vi "autonSample.vi"(0 "Auton Array":dbl[][](array[numeric]), 5 "MeasuredHeading":dbl, 9 "EncoderDistance":dbl) -> (4 "Left Drive":dbl(knob) scale=-1.0..1.0, 6 "Right Drive":dbl(knob) scale=-1.0..1.0, 10 "Turret Rotation":dbl, 14 "Feeder motor":dbl, 15 "Shooter motor output":dbl)   [LabVIEW 2011]
uses:
  Robot Global Data.vi
  <vilib>/addons/control/pid/NI_PID_pid.lvlib
  <vilib>/addons/control/pid/pid.llb/PID (DBL).vi
panel:
  out "Tzero":i64
  out "AccumDist":dbl
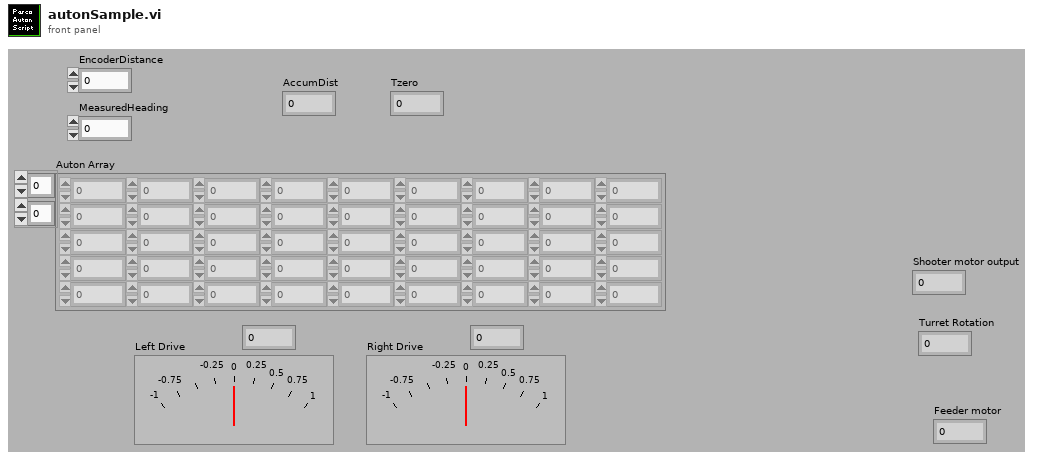
[diagram p1: front panel]
types:
  T1 = cluster{"proportional gain (Kc)":dbl, "integral time (Ti, min)":dbl, "derivative time (Td, min)":dbl}
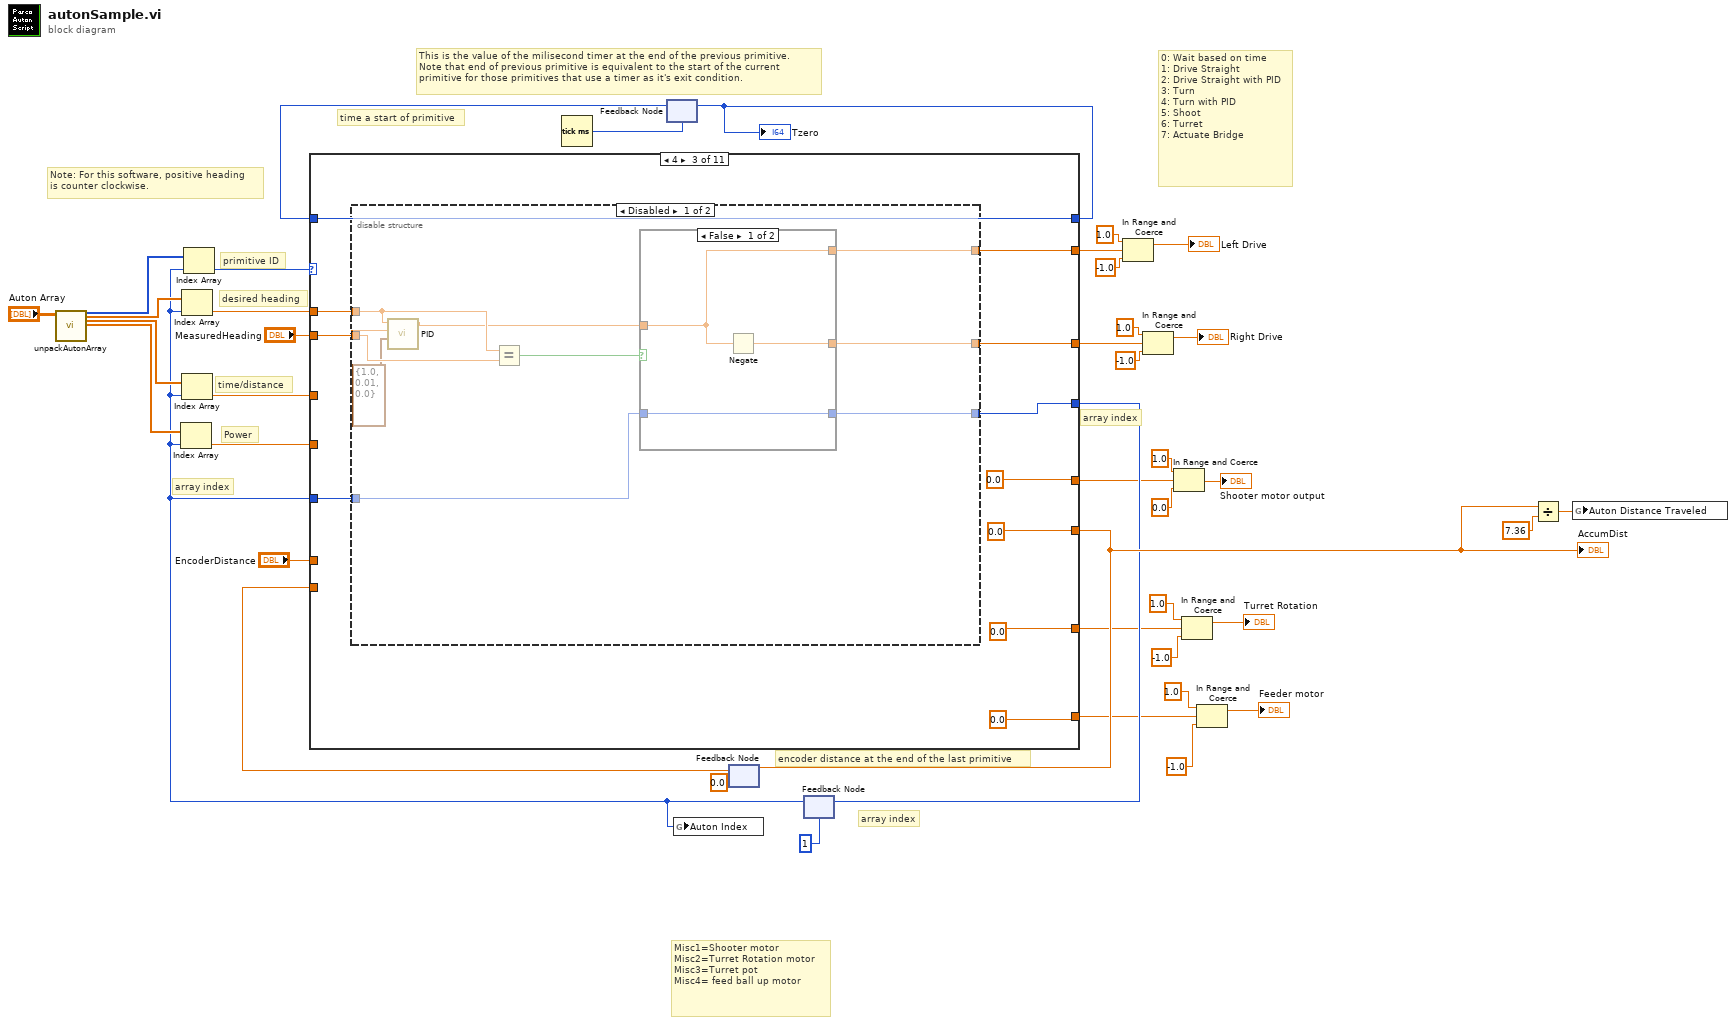
[diagram p0: block diagram]
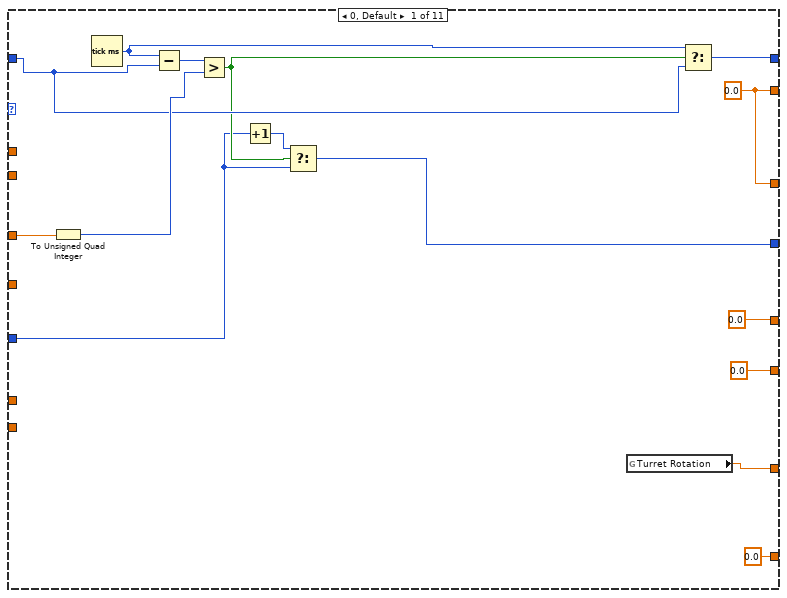
[diagram p2: hidden frame]
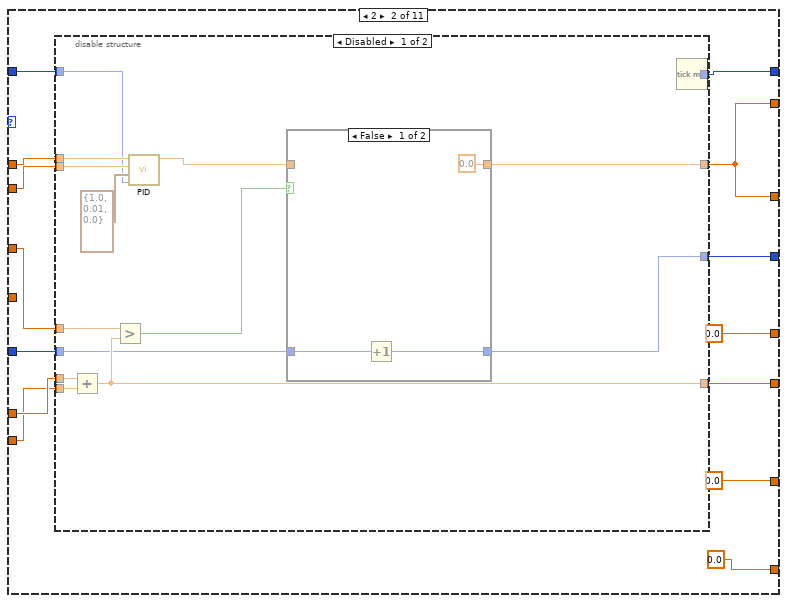
[diagram p3: hidden frame]
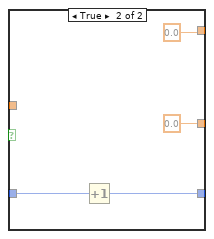
[diagram p6: hidden frame]
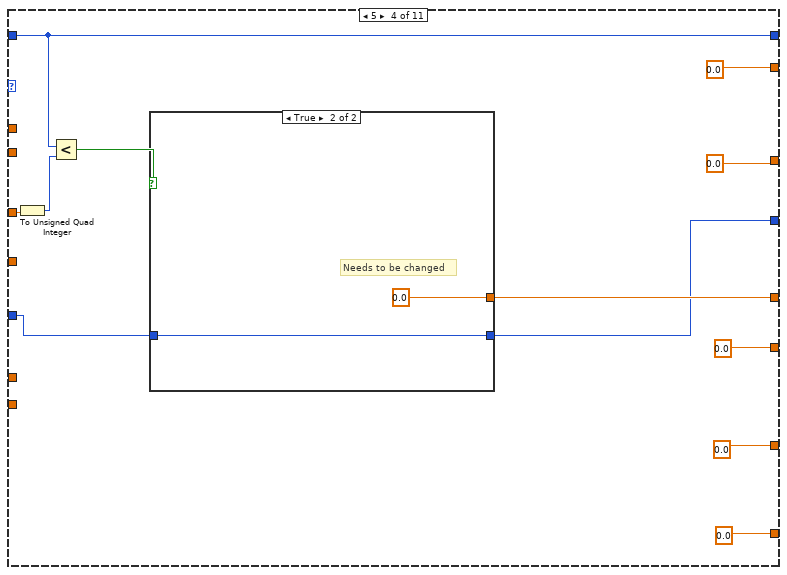
[diagram p8: hidden frame]
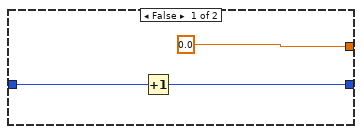
[diagram p9: hidden frame]
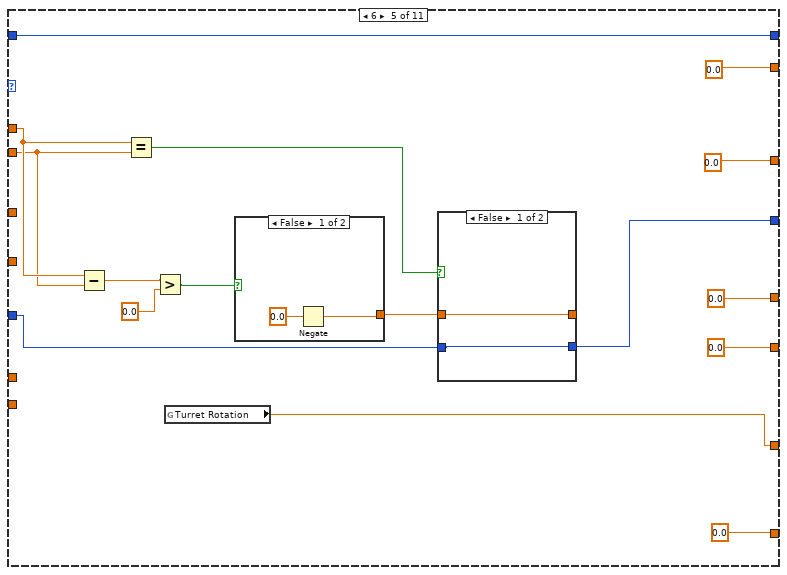
[diagram p10: hidden frame]
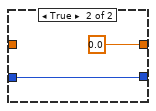
[diagram p11: hidden frame]
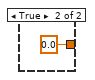
[diagram p12: hidden frame]
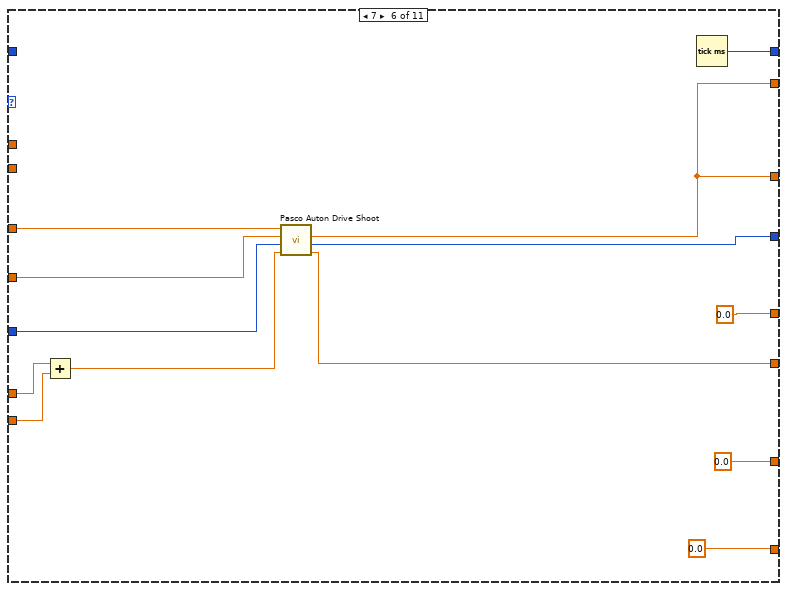
[diagram p13: hidden frame]
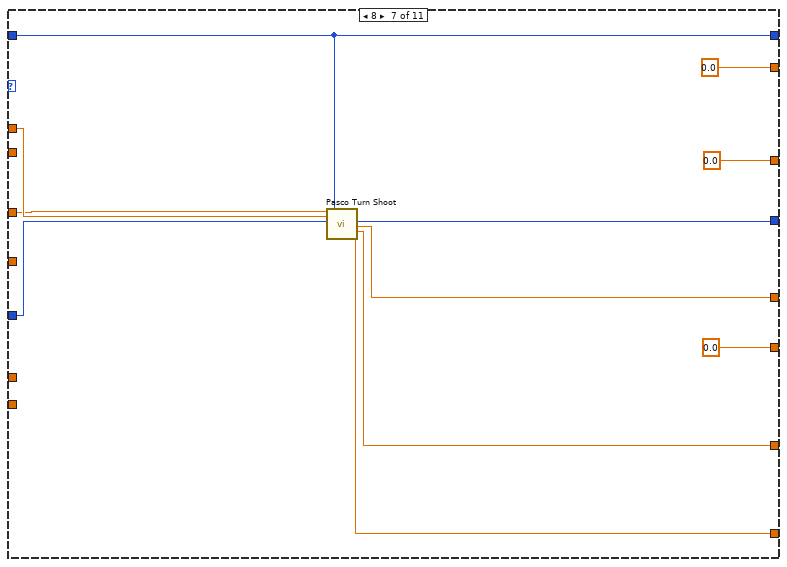
[diagram p14: hidden frame]
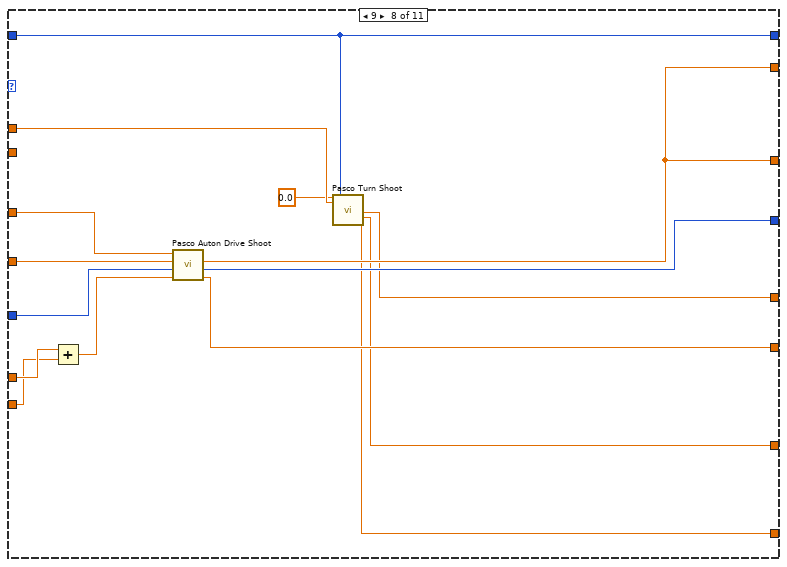
[diagram p15: hidden frame]
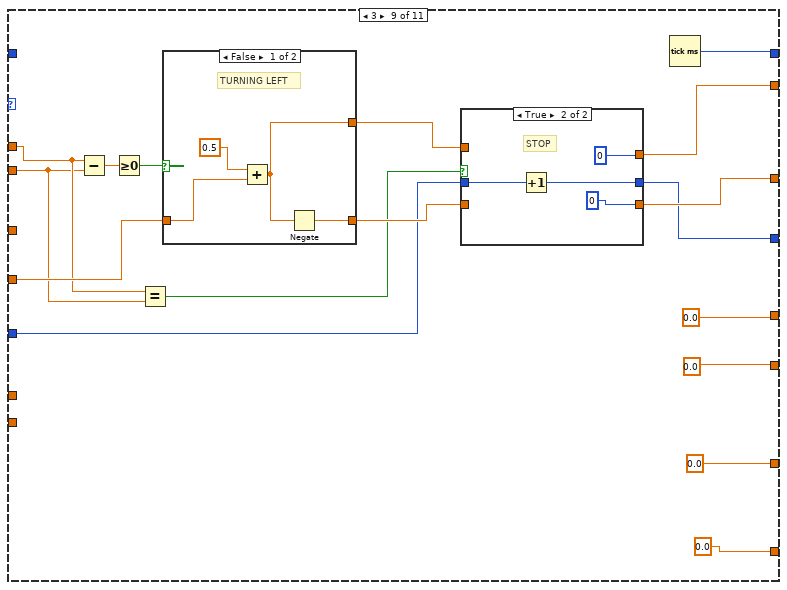
[diagram p16: hidden frame]
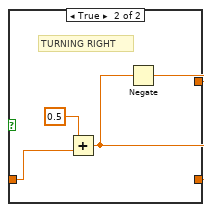
[diagram p18: hidden frame]
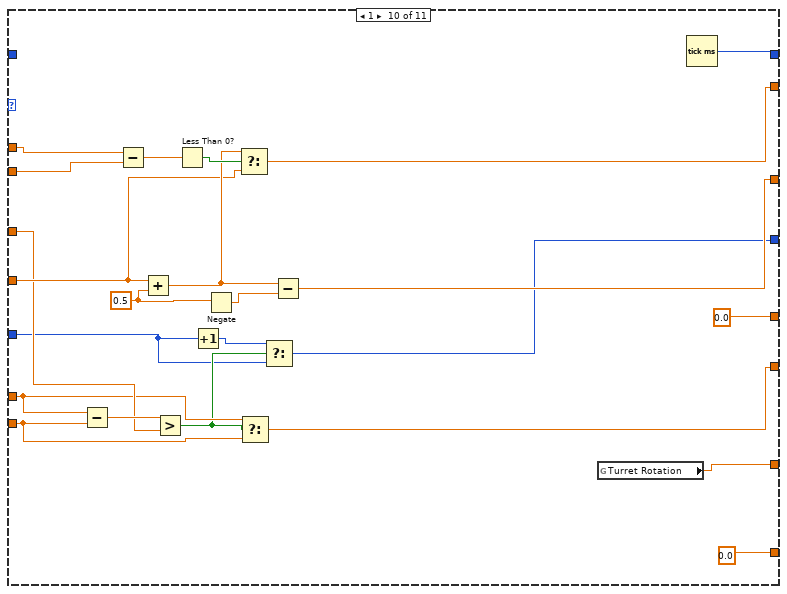
[diagram p19: hidden frame]
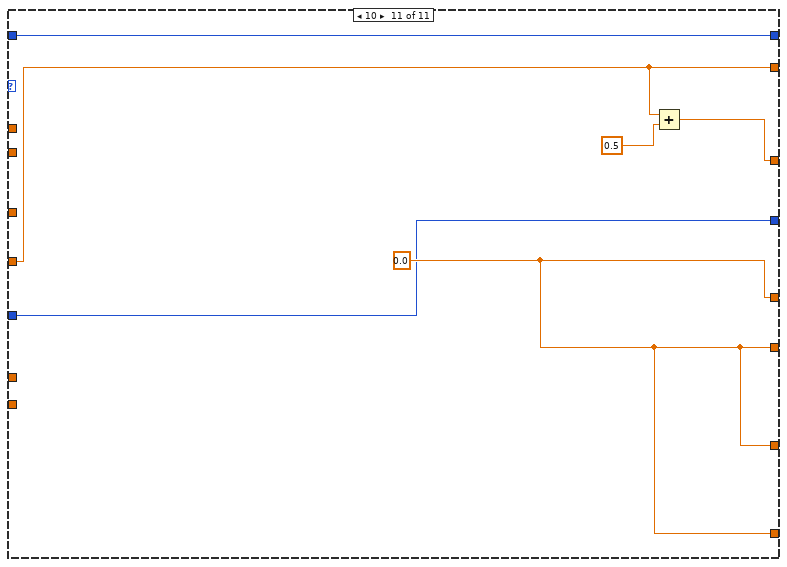
[diagram p20: hidden frame]
diagram:
  # "Misc1=Shooter motor\nMisc2=Turret Rotation motor\nMisc3=Turret pot\nMisc4= feed ball up motor"
  # "0: Wait based on time\n1: Drive Straight\n2: Drive Straight with PID\n3: Turn\n4: Turn with PID\n5: Shoot\n6: Turret\n7: Actuate Bridge"
  # "encoder distance at the end of the last primitive"
  # "Note: For this software, positive heading\nis counter clockwise."
  # "time a start of primitive"
  # "array index"
  # "array index"
  # "This is the value of the milisecond timer at the end of the previous primitive.\nNote that end of previous primitive is equivalent to the start of the current\nprimitive for those primitives that use a timer as it's exit condition."
  # "Power"
  # "array index"
  # "desired heading"
  # "primitive ID"
  # "time/distance"
  n1 = call "unpackAutonArray.vi"("all rows"="Auton Array") -> ("Primitive"=w41:i16[], "Heading"=w23:dbl[], "Distance/Time"=w24:dbl[], "Power"=w21:dbl[])  [unwired: 1 in, 22 out]
  n2 = Tick Count (ms)() -> (millisecond timer value=w35:u32)
  n3 = feedback #1(w35) -> (w39:u32)
  n4 = feedback #2(0.0 ("EncoderDistance")) -> (w20:dbl)
  n5 = feedback #3(1) -> (w2:i32)
  n6 = Index Array(array=w21, index=w2) -> (element=w37:dbl)
  n7 = Index Array(array=w23, index=w2) -> (element=w22:dbl)
  n8 = Index Array(array=w24, index=w2) -> (element=w38:dbl)
  n9 = Index Array(array=w41, index=w2) -> (element=w40:i16)
  n10 = case shown="4" w40 {
    tunnel: [w45 w64 w95 w124 w146 w163 w178 w189 w202 w230 w256] -> w15
    tunnel: w2 -> [w46 w65 w94 w125 w147 w166 w181 w194 w201 w231 w256]
    tunnel: [w57 w71 w101 w119 w145 w159 w179 w184 w208 w229 w255] -> w25
    tunnel: w39 -> [w53 w58 w101 w119 w145 _ w179 w184 _ _ w255]
    tunnel: w38 -> [w55 w67 _ w129 _ w170 w175 w196 _ w238 _]
    tunnel: w22 -> [_ w59 w91 _ w150 _ w180 w188 w210 w249 _]
    tunnel: [w44 w66 w96 0.0 0.0 w164 0.0 w187 w204 w240 w253] -> w33
    tunnel: [w44 w66 w97 0.0 0.0 w164 0.0 w187 w207 w242 w252] -> w26
    tunnel: w37 -> [_ _ _ _ _ w165 _ w195 w212 w241 w253]
    tunnel: "EncoderDistance" -> [_ w70 _ _ _ w169 _ w193 _ w237 _]
    tunnel: "MeasuredHeading" -> [_ w60 w92 _ w136 _ _ _ w209 w248 _]
    tunnel: [0.0 ("Encoder total") w68 0.0 0.0 0.0 w162 0.0 w190 0.0 w234 w257] -> w17
    tunnel: w20 -> [_ w69 _ _ _ w168 _ w192 _ w236 _]
    tunnel: [0.0 ("Misc1  OUT") 0.0 0.0 w126 0.0 0.0 ("Misc1  OUT") w177 w186 0.0 0.0 w257] -> w11
    tunnel: [w43 0.0 0.0 0.0 w135 0.0 ("Misc1  OUT") w176 w185 0.0 w235 w257] -> w7
    tunnel: [0.0 ("Misc4 OUT") 0.0 0.0 0.0 0.0 0.0 w171 w182 0.0 0.0 w257] -> w3
    frame 0, Default {
      w44 = 0.0 ("Numeric")
      n11 = To Unsigned Quad Integer(1:w55) -> (0:w54:u64)
      n12 = Tick Count (ms)() -> (millisecond timer value=w52:u32)
      n13 = Subtract(x=w52, y=w53) -> (x-y=w56:u32)
      n14 = Greater?(x=w56, y=w54) -> (0:w48:bool)
      n15 = Increment(x=w46) -> (x+1=w47:i32)
      n16 = Select(t=w47, s=w48, f=w46) -> (s? t:f=w45:i32)
      n17 = global read "Robot Global Data.vi" "Turret Rotation"() -> (w43:dbl)
      n18 = Select(t=w52, s=w48, f=w53) -> (s? t:f=w57:u32)
    }
    frame 2 {
      n19 = disable-structure shown="Disabled" {
        disable-tunnel: [w85 _] -> w71
        disable-tunnel: w70 -> [w84 _]
        disable-tunnel: w69 -> [w83 _]
        disable-tunnel: [w82 _] -> w68
        disable-tunnel: w67 -> [w81 _]
        disable-tunnel: [w79 _] -> w66
        disable-tunnel: w65 -> [w78 _]
        disable-tunnel: [w77 _] -> w64
        disable-tunnel: w60 -> [w74 _]
        disable-tunnel: w59 -> [w73 _]
        disable-tunnel: w58 -> [w72 _]
        frame Disabled {
          n20 = Add(x=w84, y=w83) -> (x+y=w82:dbl)
          n21 = Greater?(x=w81, y=w82) -> (0:w80:bool)
          n22 = call-poly <vilib>:"PID.vi"("dt (s)"=w72, "PID gains"=T1 {"proportional gain (Kc)"=1.0, "integral time (Ti, min)"=0.01, "derivative time (Td, min)"=0.0}, "process variable"=w74, "setpoint"=w73) -> ("output"=w76:dbl)  [unwired: 6 in, 1 out]
          n23 = case shown="False" w80 {
            tunnel: [0.0 w90] -> w79
            tunnel: w76 -> [_ w90]
            tunnel: w78 -> [w88 w89]
            tunnel: [w87 w89] -> w77
            frame False {
              n24 = Increment(x=w88) -> (x+1=w87:i32)
            }
            frame True {
            }
          }
          n25 = Tick Count (ms)() -> (millisecond timer value=w85:u32)
        }
        frame Enabled {
        }
      }
    }
    frame 4 {
      n26 = disable-structure shown="Disabled" {
        disable-tunnel: [w110 _] -> w97
        disable-tunnel: [w109 _] -> w96
        disable-tunnel: [w108 _] -> w95
        disable-tunnel: w94 -> [w107 _]
        disable-tunnel: w92 -> [w105 _]
        disable-tunnel: w91 -> [w104 _]
        frame Disabled {
          n27 = call-poly <vilib>:"PID.vi"("PID gains"=T1 {"proportional gain (Kc)"=1.0, "integral time (Ti, min)"=0.01, "derivative time (Td, min)"=0.0}, "process variable"=w105, "setpoint"=w104) -> ("output"=w103:dbl)  [unwired: 7 in, 1 out]
          n28 = Equal?(x=w104, y=w105) -> (x = y?=w106:bool)
          n29 = case shown="False" w106 {
            tunnel: w103 -> [w112 _]
            tunnel: [w113 0.0] -> w110
            tunnel: [w112 0.0] -> w109
            tunnel: [w111 w116] -> w108
            tunnel: w107 -> [w111 w117]
            frame False {
              n30 = Negate(x=w112) -> (-x=w113:dbl)
            }
            frame True {
              n31 = Increment(x=w117) -> (x+1=w116:i32)
            }
          }
        }
        frame Enabled {
        }
      }
    }
    frame 5 {
      n32 = To Unsigned Quad Integer(1:w129) -> (0:w127:u64)
      n33 = Less?(x=w119, y=w127) -> (x < y?=w128:bool)
      n34 = case shown="True" w128 {
        tunnel: [0.0 0.0] -> w126
        tunnel: w125 -> [w131 w134]
        tunnel: [w130 w134] -> w124
        frame False {
          n35 = Increment(x=w131) -> (x+1=w130:i32)
        }
        frame True {
          # "Needs to be changed"
        }
      }
    }
    frame 6 {
      n36 = Subtract(x=w150, y=w136) -> (x-y=w138:dbl)
      n37 = Equal?(x=w150, y=w136) -> (x = y?=w149:bool)
      n38 = Greater?(x=w138, y=0.0) -> (0:w139:bool)
      n39 = global read "Robot Global Data.vi" "Turret Rotation"() -> (w135:dbl)
      n40 = case shown="False" w139 {
        tunnel: [w156 0.0] -> w148
        frame False {
          n41 = Negate(x=0.0) -> (-x=w156:dbl)
        }
        frame True {
        }
      }
      n42 = case shown="False" w149 {
        tunnel: [w152 0.0] -> _
        tunnel: w148 -> [w152 _]
        tunnel: w147 -> [w151 w154]
        tunnel: [w151 w154] -> w146
        frame False {
        }
        frame True {
        }
      }
    }
    frame 7 {
      n43 = Add(x=w169, y=w168) -> (x+y=w167:dbl)
      n44 = call "Pasco Auton Drive Shoot.vi"("Encoder total"=w167, "Array"=w166, "Power"=w165, "time/distance"=w170) -> ("Encoder total"=w162:dbl, "Array Out"=w163:i32, "Power"=w164:dbl)  [unwired: 5 in]
      n45 = Tick Count (ms)() -> (millisecond timer value=w159:u32)
    }
    frame 8 {
      n46 = call "Pasco Turn Shoot.vi"("time/distance"=w175, "desired heading"=w180, "array index"=w181, "primitive time"=w179) -> ("array index"=w178:i32, "Misc1  OUT"=w177:dbl, "Misc2 OUT"=w176:dbl, "Misc4 OUT"=w171:dbl)  [unwired: 12 in]
    }
    frame 9 {
      n47 = Add(x=w193, y=w192) -> (x+y=w191:dbl)
      n48 = call "Pasco Auton Drive Shoot.vi"("Encoder total"=w191, "Array"=w194, "Power"=w195, "time/distance"=w196) -> ("Encoder total"=w190:dbl, "Array Out"=w189:i32, "Power"=w187:dbl)  [unwired: 5 in]
      n49 = call "Pasco Turn Shoot.vi"("time/distance"=0.0, "desired heading"=w188, "primitive time"=w184) -> ("Misc1  OUT"=w186:dbl, "Misc2 OUT"=w185:dbl, "Misc4 OUT"=w182:dbl)  [unwired: 13 in, 1 out]
    }
    frame 3 {
      n50 = Subtract(x=w210, y=w209) -> (x-y=w213:dbl)
      n51 = Greater Or Equal To 0?(x=w213) -> (x >= 0?=w211:bool)
      n52 = Equal?(x=w210, y=w209) -> (x = y?=w203:bool)
      n53 = case shown="False" w211 {
        tunnel: w212 -> [w223 w225]
        tunnel: [w221 w227] -> w205
        tunnel: [w222 w226] -> w206
        frame False {
          # "TURNING LEFT"
          n54 = Add(x=0.5, y=w223) -> (x+y=w221:dbl)
          n55 = Negate(x=w221) -> (-x=w222:dbl)
        }
        frame True {
          # "TURNING RIGHT"
          n56 = Add(x=0.5, y=w225) -> (x+y=w226:dbl)
          n57 = Negate(x=w226) -> (-x=w227:dbl)
        }
      }
      n58 = case shown="True" w203 {
        tunnel: w201 -> [w216 w220]
        tunnel: [w216 w219] -> w202
        tunnel: [w215 0] -> w207
        tunnel: w206 -> [w215 _]
        tunnel: [w214 0] -> w204
        tunnel: w205 -> [w214 _]
        frame False {
          # "DRIVE"
        }
        frame True {
          # "STOP"
          n59 = Increment(x=w220) -> (x+1=w219:i32)
        }
      }
      n60 = Tick Count (ms)() -> (millisecond timer value=w208:u32)
    }
    frame 1 {
      w244 = 0.5 ("y")
      n61 = Subtract(x=w237, y=w236) -> (x-y=w239:dbl)
      n62 = Subtract(x=w249, y=w248) -> (x-y=w247:dbl)
      n63 = Add(x=w241, y=w244) -> (x+y=w245:dbl)
      n64 = Greater?(x=w239, y=w238) -> (0:w233:bool)
      n65 = Less Than 0?(x=w247) -> (x < 0?=w246:bool)
      n66 = Increment(x=w231) -> (x+1=w232:i32)
      n67 = Negate(x=w244) -> (-x=w243:dbl)
      n68 = Select(t=w245, s=w246, f=w241) -> (s? t:f=w240:dbl)
      n69 = Select(t=w237, s=w233, f=w236) -> (s? t:f=w234:dbl)
      n70 = Select(t=w232, s=w233, f=w231) -> (s? t:f=w230:i32)
      n71 = Subtract(x=w245, y=w243) -> (x-y=w242:dbl)
      n72 = global read "Robot Global Data.vi" "Turret Rotation"() -> (w235:dbl)
      n73 = Tick Count (ms)() -> (millisecond timer value=w229:u32)
    }
    frame 10 {
      w257 = 0.0
      n74 = Add(x=w253, y=0.5 ("x+y")) -> (x+y=w252:dbl)
    }
  }
  "AccumDist" <- w17
  "Tzero" <- w25
  n75 = feedback-in #1(w25) -> ()
  n76 = global write "Robot Global Data.vi" "Auton Index"(w2) -> ()
  n77 = feedback-in #2(w17) -> ()
  n78 = feedback-in #3(w15) -> ()
  n79 = In Range and Coerce(upper limit=1.0, x=w33, lower limit=-1.0) -> (coerced(x)=→"Left Drive":dbl)  [unwired: 1 out]
  n80 = In Range and Coerce(upper limit=1.0, x=w26, lower limit=-1.0) -> (coerced(x)=→"Right Drive":dbl)  [unwired: 1 out]
  n81 = In Range and Coerce(upper limit=1.0, x=w11, lower limit=0.0) -> (coerced(x)=→"Shooter motor output":dbl)  [unwired: 1 out]
  n82 = In Range and Coerce(upper limit=1.0, x=w7, lower limit=-1.0) -> (coerced(x)=→"Turret Rotation":dbl)  [unwired: 1 out]
  n83 = In Range and Coerce(upper limit=1.0, x=w3, lower limit=-1.0) -> (coerced(x)=→"Feeder motor":dbl)  [unwired: 1 out]
  n84 = Divide(x=w17, y=7.36) -> (x/y=w1:dbl)
  n85 = global write "Robot Global Data.vi" "Auton Distance Traveled"(w1) -> ()
